vi "Random_box.vi"(8 "Error In":errorcluster) -> (0 "Error Out":errorcluster, 3 "Task Out":refnum<k21>)   [LabVIEW 2014]
uses:
  <vilib>/DAQmx/create/channels.llb/DAQmx Create Channel (AO-Voltage-Basic).vi
panel:
  in  "Physical Channels":tag="Dev3/ao0"
  in  "Max V":dbl=5.0
  in  "Min V":dbl
  # "A Random System"
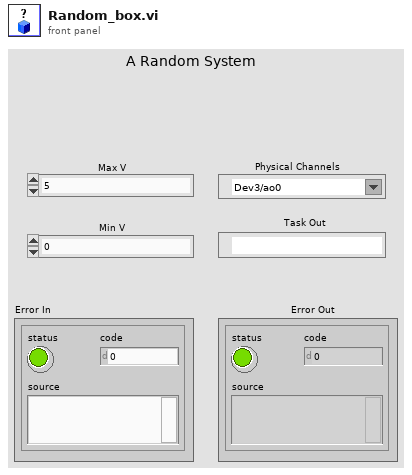
[diagram p1: front panel]
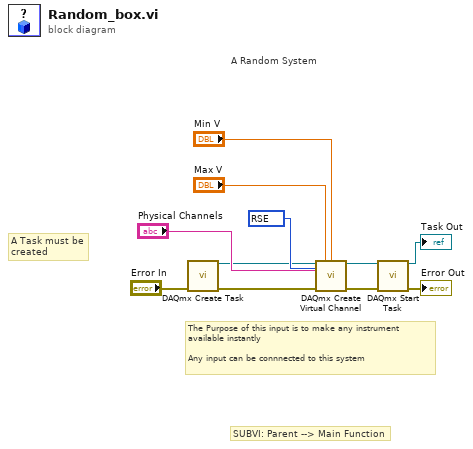
[diagram p0: block diagram]
diagram:
  w10 = 10083 items=["default"=-1, "RSE"=10083, "NRSE"=10078, "Differential"=10106, "Pseudodifferential"=12529] ("motor read")
  # "A Task must be \ncreated"
  # "SUBVI: Parent --> Main Function"
  # "The Purpose of this input is to make any instrument\navailable instantly\n\nAny input can be connnected to this system"
  # "A Random System"
  n1 = call <vilib>:"DAQmx Create Task.vi"("error in"="Error In") -> ("task out"=w6:refnum<k21>, "error out"=w7:errorcluster)  [unwired: 13 in]
  n2 = call-poly <vilib>:"DAQmx Create Virtual Channel.vi"("task in"=w6, "maximum value"="Max V", "minimum value"="Min V", "output terminal configuration"=w10, "physical channels"="Physical Channels", "error in"=w7) -> ("task out"=w5:refnum<k21>, "error out"=w4:errorcluster)  [unwired: 8 in]
  n3 = call <vilib>:"DAQmx Start Task.vi"("task/channels in"=w5, "error in"=w4) -> ("task out"=→"Task Out":refnum<k21>, "error out"=→"Error Out":errorcluster)  [unwired: 12 in]
